vi "ASYNC_Adam_server.vi"(3 "Values":dbl[](array[numeric]) format="%.2f", 4 "Client Name":string="G3_3 HD", 5 "Channel Names":string[](array[string])) -> (0 "Scan Comments":string[](array[string]), 2 "Calibrated Units":dbl[](array[numeric]) format="%.2f")   [LabVIEW 2016]
uses:
  ADAM Client/Sub VIs/ADAM Controls/Channel_State.ctl
  ADAM Client/Sub VIs/ADAM Controls/Update_scan_value.ctl
  Anemometry/Anemometry Sub Vis/Globals/Preference_global.vi
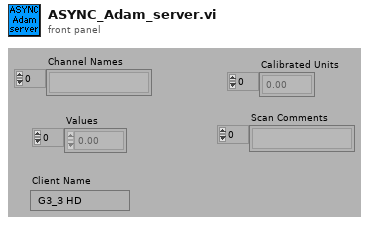
[diagram p1: front panel]
types:
  T1 = typedef "Channel_State.ctl" = enum16{"On", "Off", "Always On", "Always Off"}
  T2 = enum16{"Append to Global", "Read Global then Clear"}
  T3 = typedef "Update_scan_value.ctl" = cluster{"Channel Name":string, "New Value":dbl}
  T4 = typedef "Ch_description_ADAM.ctl" = cluster{"Ch Name":string, "Type":T5, "Function":T6, "Ch State":T1, "Calibration type":T7, "A":dbl, "B":dbl, "C":dbl, "D":dbl, "Comments":string, "Address":T8, "String":string, "Duty":u16}
  T5 = typedef "Module_type_ADAM.ctl" = string
  T6 = typedef "Function_ADAM.ctl" = enum16{"Analogue Input", "Digital Input", "Event counter", "Event rate", "Analogue Output", "Digital Output", "Relay Output"}
  T7 = typedef "Calib_type_ADAM.ctl" = string
  T8 = typedef "Address.ctl" = cluster{"Main":i32, "Ch.":i32, "Sub":i32, "Port Name":string}
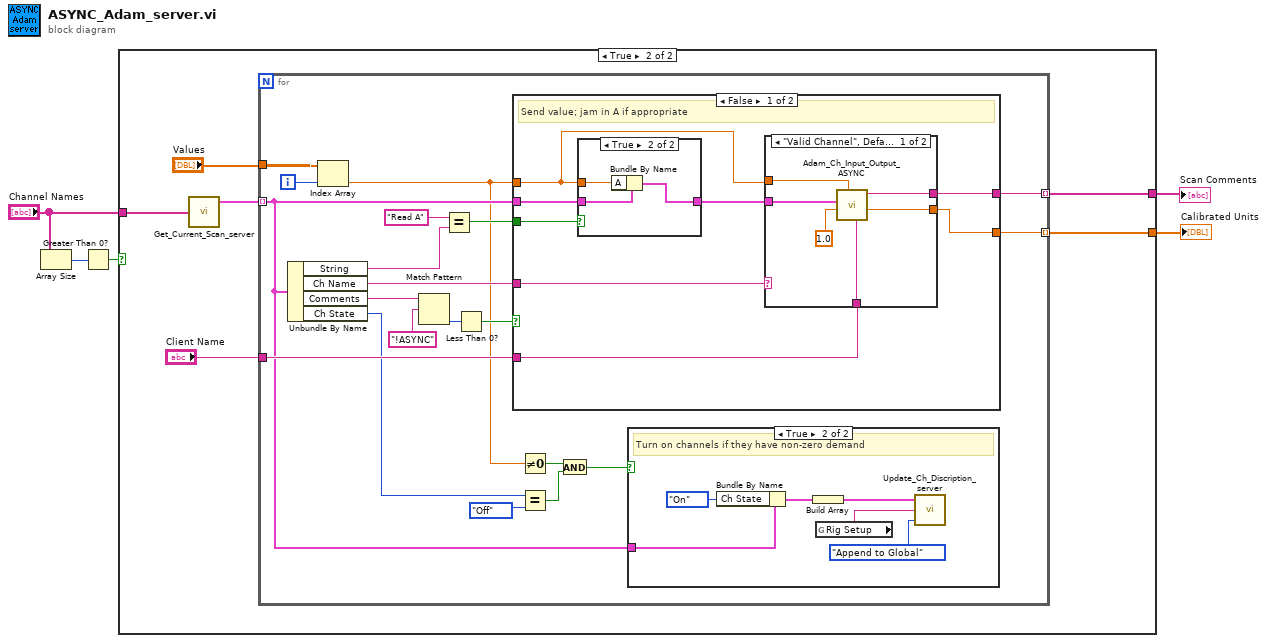
[diagram p0: block diagram]
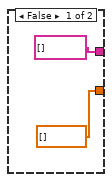
[diagram p2: hidden frame]
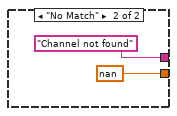
[diagram p5: hidden frame]
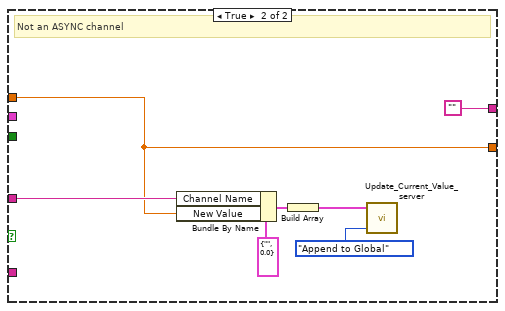
[diagram p6: hidden frame]
diagram:
  n1 = Array Size(array="Channel Names") -> (size(s)=w2:i32)
  n2 = Greater Than 0?(x=w2) -> (x > 0?=w1:bool)
  n3 = case shown="True" w1 {
    tunnel: "Channel Names" -> [_ w13]
    tunnel: [dbl[] [] w9] -> w5
    tunnel: [string[] [] w8] -> w4
    frame False {
    }
    frame True {
      n4 = call "Get_Current_Scan_server.vi"("Desired Channels"=w13) -> ("Ch Description Array"=w11:T4[])  [unwired: 2 out]
      n5 = for {
        tunnel: w11 -> [w18] mode=indexing
        tunnel: "Values" -> [w30]
        tunnel: [w33] -> w8 mode=indexing
        tunnel: [w32] -> w9 mode=indexing
        tunnel: "Client Name" -> [w29]
        i -> [w31]
        n6 = Unbundle By Name(w18) -> ("String"=w26:string, "Ch Name"=w25:string, "Comments"=w23:string, "Ch State"=w19:T1)
        n7 = Index Array(array=w30, index=w31) -> (element=w17:dbl)
        n8 = Match Pattern(string=w23, regular expression="!ASYNC" ("String to match")) -> (offset past match=w22:i32)  [unwired: 4 out]
        n9 = Equal?(x="Read A", y=w26) -> (x = y?=w28:bool)
        n10 = Less Than 0?(x=w22) -> (x < 0?=w21:bool)
        n11 = case shown="False" w21 {
          tunnel: [w47 ""] -> w33
          tunnel: [w46 w61] -> w32
          tunnel: w29 -> [w45 _]
          tunnel: w28 -> [w44 _]
          tunnel: w18 -> [w43 _]
          tunnel: w17 -> [w42 w61]
          tunnel: w25 -> [w40 w65]
          frame False {
            # "Send value; jam in A if appropriate"
            n12 = case shown="True" w44 {
              tunnel: w43 -> [w48 w51]
              tunnel: w42 -> [_ w50]
              tunnel: [w48 w49] -> w41
              frame False {
              }
              frame True {
                n13 = Bundle By Name(cluster=w51, "A"=w50) -> (w49:T4)
              }
            }
            n14 = case shown="\"Valid Channel\", Default" w40 {
              tunnel: [w57 "Channel not found" ("Scan comment")] -> w47
              tunnel: [w56 nan ("Calibrated units")] -> w46
              tunnel: w42 -> [w55 _]
              tunnel: w41 -> [w54 _]
              tunnel: w45 -> [w53 _]
              frame "Valid Channel", Default {
                n15 = call "Adam_Ch_Input_Output_ASYNC.vi"("Client Name"=w53, "Value to Output"=w55, "Scan Period"=1.0, "Ch Description"=w54) -> ("Calibrated units"=w56:dbl, "Scan comment"=w57:string)  [unwired: 3 in, 3 out]
              }
              frame "No Match" {
              }
            }
          }
          frame True {
            # "Not an ASYNC channel"
            n16 = Bundle By Name(cluster=T3 {"Channel Name"="", "New Value"=0.0} ("Update Scan Value Cluster"), "Channel Name"=w65, "New Value"=w61) -> (w64:T3)
            n17 = Build Array(w64) -> (w63:T3[])
            n18 = call "Update_Current_Value_server.vi"("Mode"=T2."Append to Global", "Update array in"=w63) -> ()  [unwired: 1 in, 1 out]
          }
        }
        n19 = Not Equal To 0?(x=w17) -> (x != 0?=w16:bool)
        n20 = Equal?(x=w19, y=Channel_State."Off" ("Ch State")) -> (x = y?=w15:bool)
        n21 = And(x=w16, y=w15) -> (x .and. y?=w14:bool)
        n22 = case shown="True" w14 {
          tunnel: w18 -> [_ w37]
          frame False {
          }
          frame True {
            # "Turn on channels if they have non-zero demand"
            n23 = Bundle By Name(cluster=w37, "Ch State"=Channel_State."On") -> (w35:T4)
            n24 = Build Array(w35) -> (w34:T4[])
            n25 = global read "Preference_global.vi" "Rig Setup"() -> (w38:string)
            n26 = call "Update_Ch_Discription_server.vi"("Mode"=T2."Append to Global", "Client HD name"=w38, "Channels to update In"=w34) -> ()  [unwired: 1 out]
          }
        }
      }
    }
  }
  "Calibrated Units" <- w5
  "Scan Comments" <- w4
